vi "Agilent SNA Send Pass Through Command.vi"(6 "SCPI? (F)":bool, 7 "Agilent SNA & SWP":T1, 8 "error in (no error)":errorcluster, 11 "VISA Resource Names":T2) -> (0 "error out":errorcluster, 2 "SNA Pass Through":refnum<visa-resource-name>, 3 "dup VISA Resource Names":T2)   [LabVIEW 2011]
uses:
  TypeDefs/Agilent SNA VISA.ctl
  TypeDefs/Agilent SNA Instrument Info.ctl
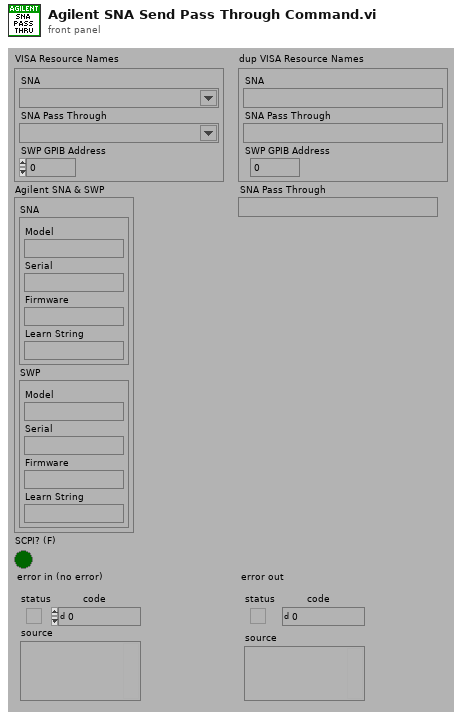
[diagram p1: front panel]
types:
  T1 = typedef "Agilent SNA Instrument Info.ctl" = cluster{"SNA":cluster{"Model":string, "Serial":string, "Firmware":string, "Learn String":string}, "SWP":cluster{"Model":string, "Serial":string, "Firmware":string, "Learn String":string}}
  T2 = typedef "Agilent SNA VISA.ctl" = cluster{"SNA":refnum<visa-resource-name>, "SNA Pass Through":refnum<visa-resource-name>, "SWP GPIB Address":i32}
  T3 = typedef "Agilent SNA SWP Model.ctl" = enum16{"Not Supported", "836XXX", "8375XX", "E82X7D"}
  T4 = typedef "Agilent SNA Model.ctl" = enum16{"Not Supported", "8757X"}
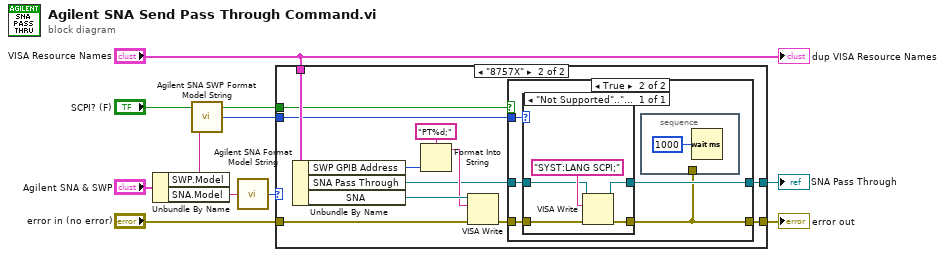
[diagram p0: block diagram]
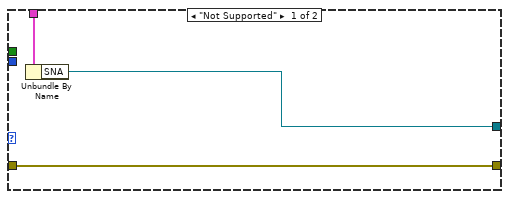
[diagram p2: hidden frame]
diagram:
  n1 = Unbundle By Name("Agilent SNA & SWP") -> ("SWP.Model"=w3:string, "SNA.Model"=w4:string)
  n2 = call "Agilent SNA SWP Format Model String.vi"("Model String"=w3) -> ("Model"=w2:T3)
  n3 = call "Agilent SNA Format Model String.vi"("Model String"=w4) -> ("Model"=w6:T4)
  n4 = case shown="\"8757X\"" w6 {
    tunnel: "error in (no error)" -> [w11 w25]
    tunnel: "VISA Resource Names" -> [w13 w24]
    tunnel: [w12 w18] -> w8
    tunnel: [w11 w17] -> w7
    tunnel: w2 -> [_ w20]
    tunnel: "SCPI? (F)" -> [_ w16]
    frame "Not Supported" {
      n5 = Unbundle By Name(w13) -> ("SNA"=w12:refnum<visa-resource-name>)
    }
    frame "8757X" {
      n6 = Unbundle By Name(w24) -> ("SWP GPIB Address"=w15:i32, "SNA Pass Through"=w14:refnum<visa-resource-name>, "SNA"=w22:refnum<visa-resource-name>)
      n7 = Format Into String(format string="PT%d;", w15) -> (resulting string=w21:string)  [unwired: 2 in, 1 out]
      n8 = VISA Write(VISA resource name=w22, write buffer=w21, error in (no error)=w25) -> (error out=w19:errorcluster)  [unwired: 2 out]
      n9 = case shown="True" w16 {
        tunnel: w20 -> [_ w32]
        tunnel: w19 -> [w27 w31]
        tunnel: [w26 w30] -> w18
        tunnel: [w27 w29] -> w17
        tunnel: w14 -> [w26 w28]
        frame False {
          # "Remain in analyzer language."
        }
        frame True {
          n10 = case shown="\"Not Supported\"..\"E82X7D\"" w32 {
            tunnel: w31 -> [w38]
            tunnel: [w36] -> w29
            tunnel: [w35] -> w30
            tunnel: w28 -> [w34]
            frame "Not Supported".."E82X7D" {
              n11 = VISA Write(VISA resource name=w34, write buffer="SYST:LANG SCPI;" ("format string"), error in (no error)=w38) -> (VISA resource name out=w35:refnum<visa-resource-name>, error out=w36:errorcluster)  [unwired: 1 out]
            }
          }
          n12 = stacked-sequence {
            tunnel: w29 -> [_]
            frame #0 {
              n13 = Wait (ms)(milliseconds to wait=u32 1000) -> ()  [unwired: 1 out]
            }
          }
        }
      }
    }
  }
  "error out" <- w7
  "SNA Pass Through" <- w8
  "dup VISA Resource Names" <- "VISA Resource Names"
